vi "Get Timeout.vi"(8 "error in (no error)":errorcluster caption="entrée d'erreur (pas d'erreur)", 11 "Class Instrument Patterm_Matching en entrée":refnum<class "Class Instrument Patterm_Matching.lvclass">) -> (0 "error out":errorcluster caption="sortie d'erreur", 2 "Timeout":u16, 3 "Class Instrument Patterm_Matching en sortie":refnum<class "Class Instrument Patterm_Matching.lvclass">)   [LabVIEW 2020, in "Library Instrument & Equipement.lvlib" / "Library Instruments.lvlib" / "Class Instrument Patterm_Matching.lvclass"]
uses:
  Class Instrument Patterm_Matching.lvclass
  Class Instrument Patterm_Matching.lvclass/Class Instrument Patterm_Matching.ctl
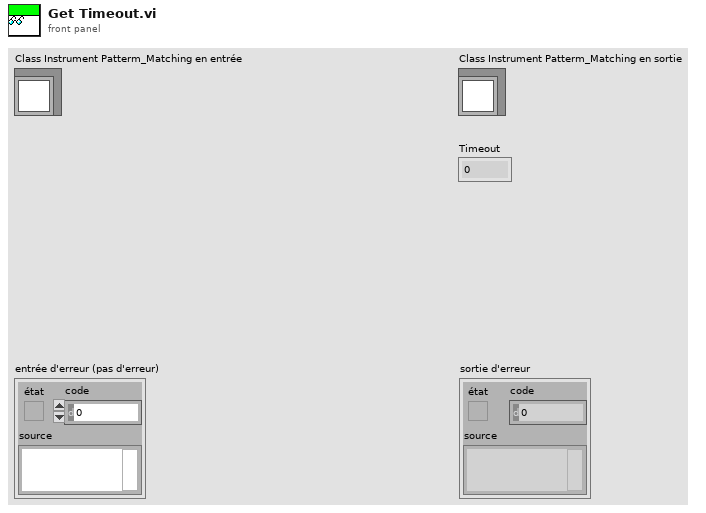
[diagram p1: front panel]
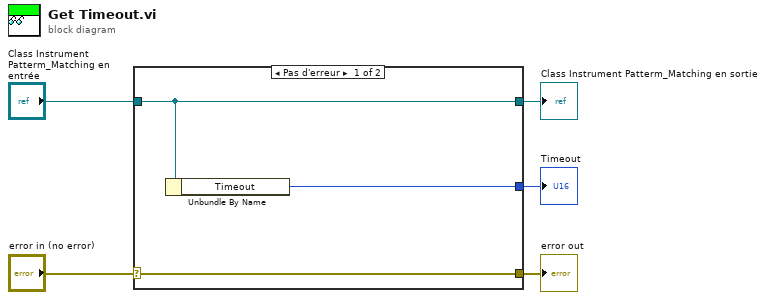
[diagram p0: block diagram]
diagram:
  n1 = case shown="Pas d'erreur" "error in (no error)" {
    selector: "error in (no error)" -> [w8 w9]
    tunnel: [w8 w9] -> w4
    tunnel: [w7 w10] -> w2
    tunnel: "Class Instrument Patterm_Matching en entrée" -> [w7 w10]
    tunnel: [w6 _] -> w1
    frame No Error {
      n2 = Unbundle By Name(w7) -> ("Timeout"=w6:u16)
    }
    frame Error {
    }
  }
  "error out" <- w4
  "Class Instrument Patterm_Matching en sortie" <- w2
  "Timeout" <- w1
